vi "Example VI for Export.vi"() -> ()   [LabVIEW 2015]
panel:
  in  "stop":bool
  out "error out":errorcluster
  in  "error in (no error)":errorcluster
  in  "String":string
  in  "Boolean":bool
  # "This is an example VI Front Panel (FP) used to export using POC"
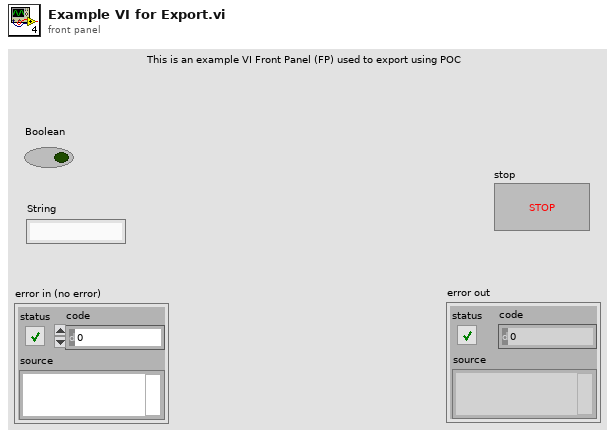
[diagram p1: front panel]
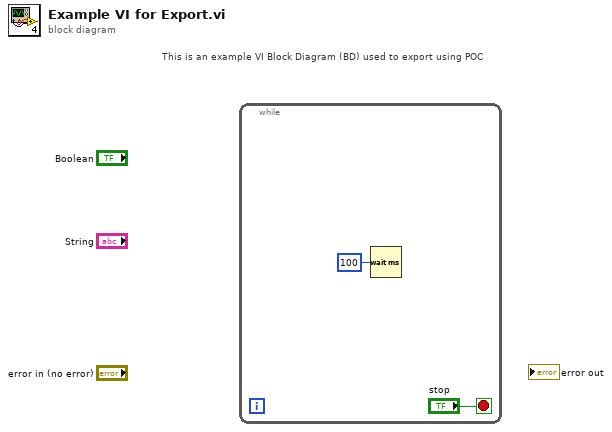
[diagram p0: block diagram]
diagram:
  # "This is an example VI Block Diagram (BD) used to export using POC"
  n1 = while {
    stop <- "stop" stop-if-true
    n2 = Wait (ms)(milliseconds to wait=u32 100) -> ()  [unwired: 1 out]
  }
